vi "MoveSinglePIMotor_C884.vi"(0 "System no.":i32=1 min=1 step=1, 1 "Axes to move":string[](array[string]), 2 "Move":dbl[](array[numeric]) format="%.6f", 5 "error in":errorcluster, 6 "Define home":bool, 7 "Move relative (-)":bool, 8 "Go home":bool, 9 "Move relative (+)":bool, 11 "Move absolute":bool, 12 "Stop refnum":refnum<vi>) -> (15 "Position":dbl[](array[numeric]) format="%.6f", 19 "error out":errorcluster)   [LabVIEW 2014]
doc: "This VI is runs in a loop until the stop button is pressed, the stop reference is TRUE or an error occures. It lets the operator set the velocity, move the connected axes to relative, absolute or to the home position, and reads the current position continuosly. The diagram shows how to combine the driver and support VIs for these tasks. Use the Help?Show Context Help menu sequence in the LabVIEW environment to display the Context Help window with the VI and control/indicator descriptions.\nRun \" XXXX_Configuration_Setup.vi\" (with XXXX being the PI product number of your system) prior to running this VI. \n\nValid for: C-843, C-843.PM, C-865, C-866, Mercury"
uses:
  C:/Users/Public/PI/GCSMergedLabVIEW/Low Level/General command.llb/Global2 (Array).vi
panel:
  in  "Clear":bool
  in  "stop":bool
  out "Conn. Axes":string[](array[string])
  # "Command move:"
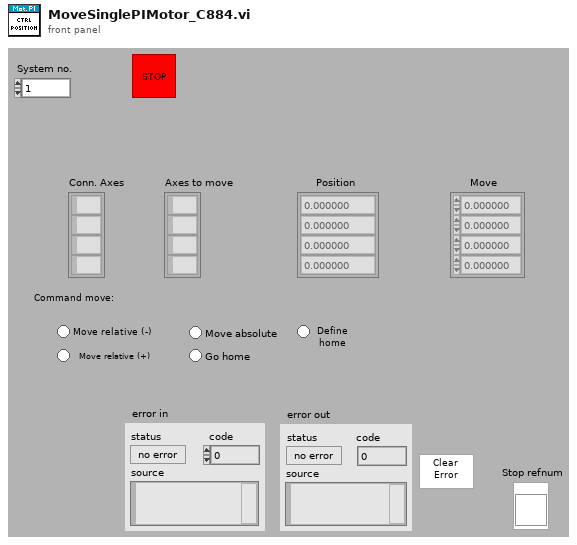
[diagram p1: front panel]
types:
  T1 = typedef "Controller names.ctl" = enum16{"None", "Analog", "C-702", "C-843", "C-843.PM", "C-844", "C-848", "C-865", "C-866", "C-867", "C-880", "C-884", "E-516", "E-517", "E-709", "E-710", "E-712", "E-725", "E-753", "E-755", "E-761", "E-816", "E-861", "E-870", "F-206", "HydraPollux", "M-840", "M-850", "M-8X0", "Mercury", "Mercury_GCS"}
  T2 = cluster{"Conn. axes":string[], "Controller name":T1}[]
  T3 = cluster{"Conn. axes":string[], "Controller name":T1}
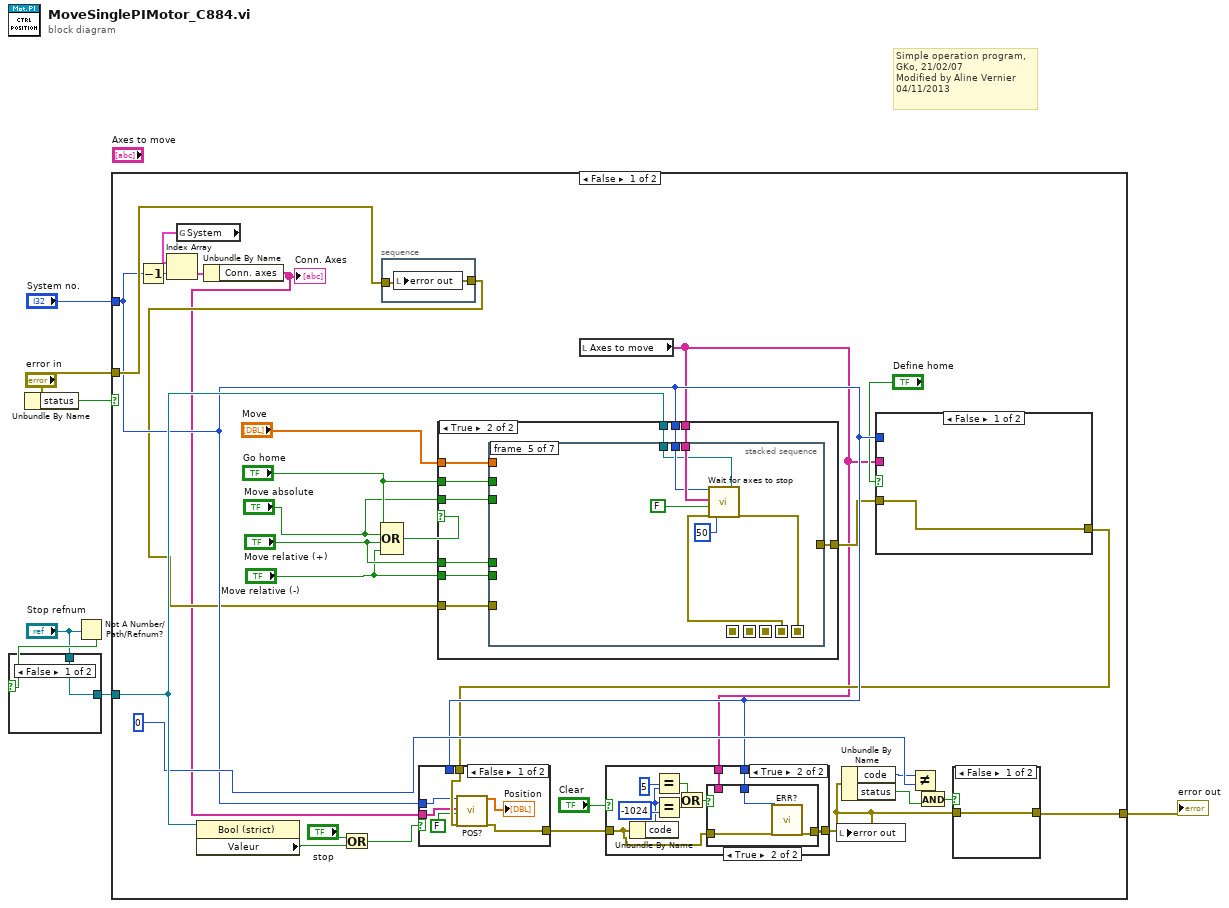
[diagram p0: block diagram]
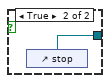
[diagram p2: hidden frame]
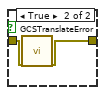
[diagram p3: hidden frame]
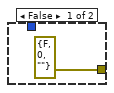
[diagram p5: hidden frame]
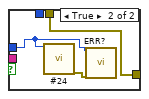
[diagram p6: hidden frame]
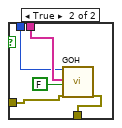
[diagram p9: hidden frame]
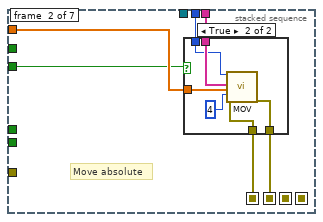
[diagram p10: hidden frame]
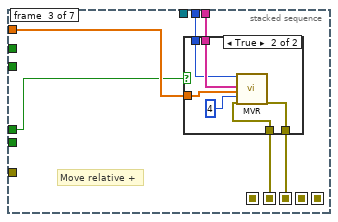
[diagram p12: hidden frame]
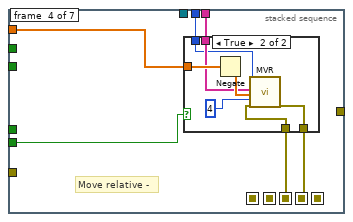
[diagram p14: hidden frame]
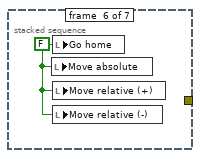
[diagram p16: hidden frame]
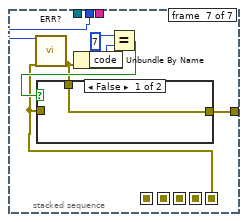
[diagram p17: hidden frame]
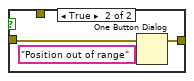
[diagram p18: hidden frame]
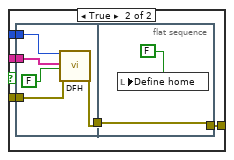
[diagram p19: hidden frame]
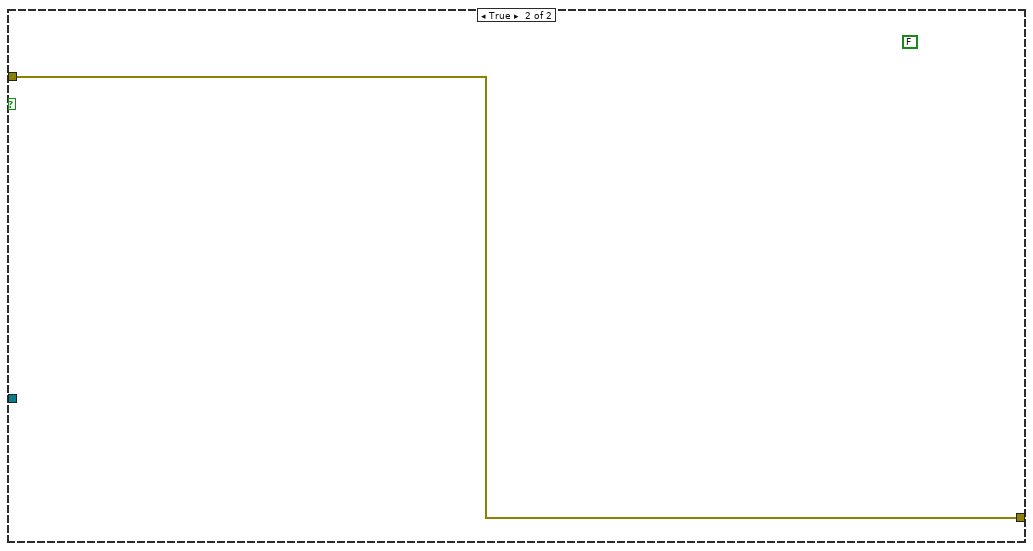
[diagram p20: hidden frame]
diagram:
  # "Simple operation program,\nGKo, 21/02/07\nModified by Aline Vernier\n04/11/2013"
  n1 = Unbundle By Name("error in") -> ("status"=w6:bool)
  n2 = Not A Number/Path/Refnum?(number/path/refnum="Stop refnum") -> (NaN/Path/Refnum?=w3:bool)
  n3 = case shown="False" w3 {
    tunnel: [w8 w9] -> w2
    tunnel: "Stop refnum" -> [w8 _]
    frame False {
    }
    frame True {
      n4 = control-ref of="stop"() -> (w9:refnum<vi>)
    }
  }
  n5 = case shown="False" w6 {
    tunnel: [w39 w161] -> w5
    tunnel: "error in" -> [w38 w161]
    tunnel: "System no." -> [w35 _]
    tunnel: w2 -> [w37 _]
    frame False {
      n6 = Decrement(x=w35) -> (x-1=w34:i32)
      n7 = global read "Global2 (Array).vi" "System"() -> (w33:T2)
      n8 = Index Array(array=w33, index=w34) -> (element=w32:T3)
      n9 = property class="Bool (strict)"(reference=w37) -> ("Valeur"=w26:bool)  [unwired: 1 in, 2 out]
      n10 = Unbundle By Name(w32) -> ("Conn. axes"=w11:string[])
      "Conn. Axes" <- w11
      n11 = Or(x="stop", y=w26) -> (x .or. y?=w12:bool)
      n12 = Compound Arithmetic op=OR("Go home", "Move absolute", "Move relative (+)", "Move relative (-)") -> (w14:bool)
      n13 = stacked-sequence {
        tunnel: w38 -> [w160]
        tunnel: [w160] -> w31
        frame #0 {
          n14 = local write "error out"(w160) -> ()
        }
      }
      n15 = local read "Axes to move"() -> (w13:string[])
      n16 = case shown="True" w14 {
        tunnel: "Go home" -> [_ w77]
        tunnel: w35 -> [_ w76]
        tunnel: w13 -> [_ w75]
        tunnel: "Move" -> [_ w74]
        tunnel: [w67 w73] -> w25
        tunnel: w37 -> [_ w72]
        tunnel: "Move absolute" -> [_ w71]
        tunnel: "Move relative (+)" -> [_ w70]
        tunnel: w31 -> [w67 w69]
        tunnel: "Move relative (-)" -> [_ w68]
        frame False {
        }
        frame True {
          n17 = stacked-sequence {
            seq-local: [w79 _ _ _ _ _ _] -> [_ w92 _ _ _ _ _]
            seq-local: [_ w90 _ _ _ _ _] -> [_ _ w103 _ _ _ _]
            seq-local: [_ _ w104 _ _ _ _] -> [_ _ _ w117 _ _ _]
            seq-local: [_ _ _ w116 _ _ _] -> [_ _ _ _ w135 _ _]
            seq-local: [_ _ _ _ w134 _ _] -> [_ _ _ _ _ _ w139]
            tunnel: w77 -> [w82 _ _ _ _ _ _]
            tunnel: w76 -> [w81 w94 w107 w120 w130 _ w140]
            tunnel: w75 -> [w80 w93 w106 w119 w131 _ _]
            tunnel: w74 -> [_ w91 w105 w118 _ _ _]
            tunnel: [_ _ _ _ _ _ w141] -> w73
            tunnel: w72 -> [_ _ _ _ w129 _ _]
            tunnel: w71 -> [_ w89 _ _ _ _ _]
            tunnel: w70 -> [_ _ w102 _ _ _ _]
            tunnel: w69 -> [w78 _ _ _ _ _ _]
            tunnel: w68 -> [_ _ _ w115 _ _ _]
            frame #0 {
              n18 = case shown="False" w82 {
                tunnel: w81 -> [_ w84]
                tunnel: w80 -> [_ w88]
                tunnel: [w83 w85] -> w79
                tunnel: w78 -> [w83 w86]
                frame False {
                }
                frame True {
                  n19 = call "GOH.vi"("System no."=w84, "GOH axes"=w88, "All axes?"=FALSE, "error in"=w86) -> ("error out"=w85:errorcluster)  [unwired: 15 in]
                }
              }
            }
            frame #1 {
              # "Move absolute"
              n20 = case shown="True" w89 {
                tunnel: w94 -> [_ w98]
                tunnel: w93 -> [_ w99]
                tunnel: w92 -> [w95 w100]
                tunnel: w91 -> [_ w96]
                tunnel: [w95 w97] -> w90
                frame False {
                }
                frame True {
                  n21 = call "MOV.vi"("System no."=w98, "Axes to move"=w99, "Position values"=w96, "No.of digits"=i16 4, "error in"=w100) -> ("error out"=w97:errorcluster)  [unwired: 14 in]
                }
              }
            }
            frame #2 {
              # "Move relative +"
              n22 = case shown="True" w102 {
                tunnel: w107 -> [_ w111]
                tunnel: w106 -> [_ w112]
                tunnel: w105 -> [_ w113]
                tunnel: [w108 w109] -> w104
                tunnel: w103 -> [w108 w110]
                frame False {
                }
                frame True {
                  n23 = call "MVR.vi"("System no."=w111, "Axes to move"=w112, "Position values"=w113, "No.of digits"=i16 4, "error in"=w110) -> ("error out"=w109:errorcluster)  [unwired: 14 in]
                }
              }
            }
            frame #3 {
              # "Move relative -"
              n24 = case shown="True" w115 {
                tunnel: w120 -> [_ w124]
                tunnel: w119 -> [_ w125]
                tunnel: w118 -> [_ w128]
                tunnel: w117 -> [w121 w123]
                tunnel: [w121 w122] -> w116
                frame False {
                }
                frame True {
                  n25 = Negate(x=w128) -> (-x=w126:dbl[])
                  n26 = call "MVR.vi"("System no."=w124, "Axes to move"=w125, "Position values"=w126, "No.of digits"=i16 4, "error in"=w123) -> ("error out"=w122:errorcluster)  [unwired: 14 in]
                }
              }
            }
            frame #4 {
              n27 = call "Wait for axes to stop.vi"("System no."=w130, "Axes to wait for"=w131, "With status bit polling?"=FALSE, "error in"=w135, "Polling cycle time, ms"=u32 50, "Stop refnum"=w129) -> ("error out"=w134:errorcluster)  [unwired: 12 in, 1 out]
            }
            frame #5 {
              w136 = FALSE ("Go home")
              n28 = local write "Move absolute"(w136) -> ()
              n29 = local write "Go home"(w136) -> ()
              n30 = local write "Move relative (+)"(w136) -> ()
              n31 = local write "Move relative (-)"(w136) -> ()
            }
            frame #6 {
              n32 = call "ERR?.vi"("System no."=w140, "error in"=w139) -> ("error out"=w138:errorcluster)  [unwired: 16 in, 1 out]
              n33 = Unbundle By Name(w138) -> ("code"=w137:i32)
              n34 = Equal?(x=7 ("y"), y=w137) -> (x = y?=w142:bool)
              n35 = case shown="False" w142 {
                tunnel: [w144 w145] -> w141
                tunnel: w139 -> [_ w145]
                tunnel: w138 -> [w144 _]
                frame False {
                }
                frame True {
                  n36 = One Button Dialog(message="Position out of range") -> ()  [unwired: 1 in, 1 out]
                }
              }
            }
          }
        }
      }
      n37 = case shown="False" "Define home" {
        tunnel: w35 -> [_ w152]
        tunnel: w13 -> [_ w151]
        tunnel: w25 -> [w147 w150]
        tunnel: [w147 w149] -> w24
        frame False {
        }
        frame True {
          n38 = flat-sequence {
            tunnel: w152 -> [w157]
            tunnel: w151 -> [w156]
            tunnel: w150 -> [w154]
            tunnel: [w153] -> w148
            tunnel: [w159] -> w149
            tunnel: w148 -> [w159]
            frame #0 {
              n39 = call "DFH.vi"("System no."=w157, "DFH axes"=w156, "All axes?"=FALSE, "error in"=w154) -> ("error out"=w153:errorcluster)  [unwired: 15 in]
            }
            frame #1 {
              n40 = local write "Define home"(FALSE ("All axes?")) -> ()
            }
          }
        }
      }
      n41 = case shown="False" w12 {
        tunnel: w35 -> [w58 w65]
        tunnel: w35 -> [_ _]
        tunnel: w24 -> [w61 w66]
        tunnel: [w62 w66] -> w22
        tunnel: w11 -> [w59 _]
        frame False {
          n42 = call "POS?.vi"("System no."=w58, "Axes to query"=w59, "All axes?"=FALSE, "error in"=w61) -> ("Position"=→"Position":dbl[], "error out"=w62:errorcluster)  [unwired: 14 in]
        }
        frame True {
          n43 = call "#24.vi"("System no."=w65) -> ("error out"=w64:errorcluster)  [unwired: 18 in]
          n44 = call "ERR?.vi"("System no."=w65, "error in"=w64) -> ()  [unwired: 16 in, 2 out]
        }
      }
      n45 = case shown="True" "Clear" {
        tunnel: [w43 w47] -> w18
        tunnel: w22 -> [w43 w44]
        tunnel: w35 -> [_ w46]
        tunnel: w13 -> [_ w45]
        frame False {
        }
        frame True {
          n46 = Unbundle By Name(w44) -> ("code"=w51:i32)
          n47 = Equal?(x=5 ("y"), y=w51) -> (x = y?=w50:bool)
          n48 = Equal?(x=w51, y=-1024) -> (x = y?=w48:bool)
          n49 = Or(x=w50, y=w48) -> (x .or. y?=w49:bool)
          n50 = case shown="True" w49 {
            tunnel: [errorcluster {"status"=FALSE, "code"=0, "source"=""} ("error out") w56] -> w47
            tunnel: w46 -> [_ w57]
            tunnel: w45 -> [_ _]
            tunnel: w44 -> [_ w55]
            frame False {
            }
            frame True {
              n51 = call "ERR?.vi"("System no."=w57, "error in"=w55) -> ("error out"=w56:errorcluster)  [unwired: 16 in, 1 out]
            }
          }
        }
      }
      n52 = local write "error out"(w18) -> ()
      n53 = Unbundle By Name(w18) -> ("code"=w21:i32, "status"=w17:bool)
      n54 = Not Equal?(x=w21, y=0 ("code")) -> (x != y?=w20:bool)
      n55 = And(x=w20, y=w17) -> (x .and. y?=w19:bool)
      n56 = case shown="False" w19 {
        tunnel: w18 -> [w40 w42]
        tunnel: [w40 w41] -> w39
        frame False {
        }
        frame True {
          n57 = call "GCSTranslateError.vi"("error in"=w42) -> ("error out"=w41:errorcluster)  [unwired: 16 in, 2 out]
        }
      }
    }
    frame True {
      (unwired) FALSE ("stop")
    }
  }
  "error out" <- w5
